vi "Data Access.vi"(9 "Time Out In ms":i32=-1, 11 "Circular Buffer 1D U16 DVR Queue in":refnum<class "Circular Buffer 1D U16 DVR Queue.lvclass">) -> (1 "Time Out":bool, 2 "Data Out":u16[](array[numeric]), 3 "Circular Buffer 1D U16 DVR Queue out":refnum<class "Circular Buffer 1D U16 DVR Queue.lvclass">)   [LabVIEW 2024, in "Circular Buffer 1D U16 DVR Queue.lvclass"]
uses:
  Circular Buffer 1D U16 DVR Queue.lvclass
  Circular Buffer 1D U16 DVR Queue.lvclass/Circular Buffer 1D U16 DVR Queue.ctl
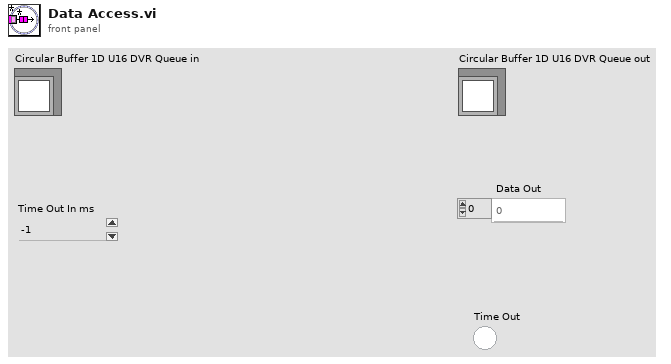
[diagram p1: front panel]
types:
  T1 = typedef "1D U16 DVR Queue.ctl" = refnum<queue>
  T2 = typedef "1D U16 DVR.ctl" = refnum<data-value>
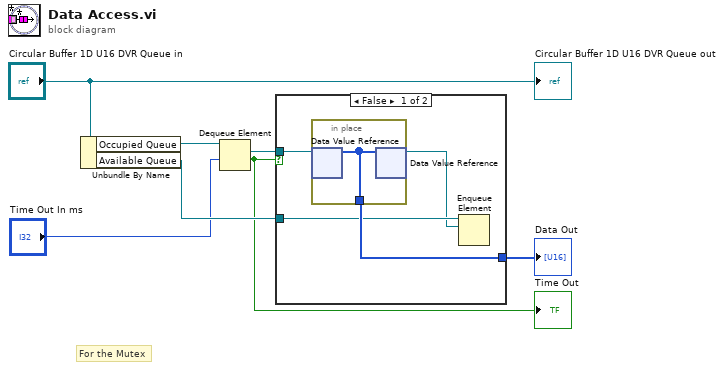
[diagram p0: block diagram]
diagram:
  # "For the Mutex"
  n1 = Unbundle By Name("Circular Buffer 1D U16 DVR Queue in") -> ("Occupied Queue"=w5:T1, "Available Queue"=w3:T1)
  n2 = Dequeue Element(queue=w5, timeout in ms (-1)="Time Out In ms") -> (element=w4:T2, timed out?=w2:bool)  [unwired: 1 in, 2 out]
  "Time Out" <- w2
  n3 = case shown="False" w2 {
    tunnel: [w11 _] -> w6
    tunnel: w4 -> [w10 _]
    tunnel: w3 -> [w9 _]
    frame False {
      n4 = in-place {
        in-place-border: [w12] -> w11
        n5 = in-place-dvr #1(w10) -> (w12:u16[])  [unwired: 1 out]
        n6 = in-place-dvr #1(w12) -> (w8:T2)  [unwired: 1 out]
      }
      n7 = Enqueue Element(queue=w9, element=w8) -> ()  [unwired: 2 in, 3 out]
    }
    frame True {
    }
  }
  "Data Out" <- w6
  "Circular Buffer 1D U16 DVR Queue out" <- "Circular Buffer 1D U16 DVR Queue in"
